vi "set_LimitSwitches.vi"(8 "error in (no error)":errorcluster caption="错误输入（无错误）", 10 "LimitSwitches":refnum<class "LimitSwitch.lvclass">[](array[class]), 11 "OneMotion输入":refnum<class "OneMotion.lvclass">) -> (0 "error out":errorcluster caption="错误输出", 3 "OneMotion输出":refnum<class "OneMotion.lvclass">)   [LabVIEW 2016, in "MotionControl.lvlib" / "OneMotion.lvclass"]
uses:
  <userlib>/MotionControl/OneMotion/OneMotion.lvclass
  <userlib>/MotionControl/LimitSwitch/LimitSwitch.lvclass
  <userlib>/MotionControl/OneMotion/OneMotion.lvclass/OneMotion.ctl
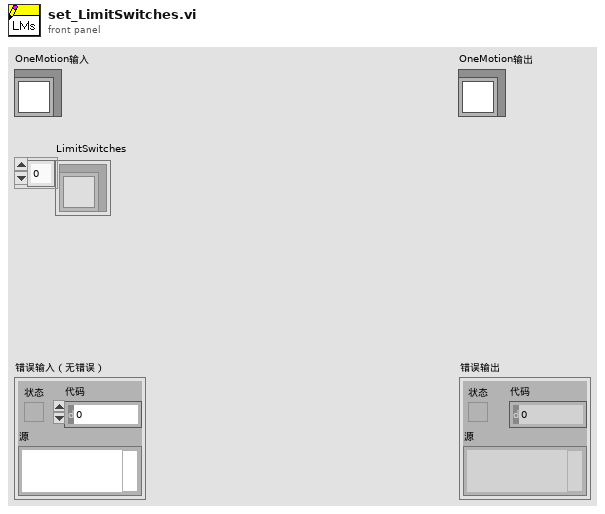
[diagram p1: front panel]
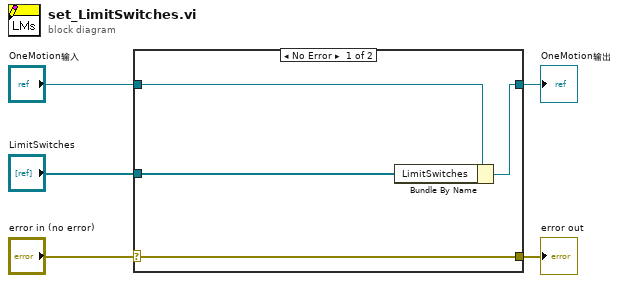
[diagram p0: block diagram]
diagram:
  n1 = case shown="No Error" "error in (no error)" {
    selector: "error in (no error)" -> [w9 w10]
    tunnel: [w9 w10] -> w4
    tunnel: [w7 w11] -> w2
    tunnel: "OneMotion输入" -> [w8 w11]
    tunnel: "LimitSwitches" -> [w6 _]
    frame No Error {
      n2 = Bundle By Name(cluster=w8, "LimitSwitches"=w6) -> (w7:refnum<class "OneMotion.lvclass">)
    }
    frame Error {
    }
  }
  "error out" <- w4
  "OneMotion输出" <- w2
